vi "CreateARtoolkitHeader.vi"(8 "error in (no error)":errorcluster) -> (0 "error out":errorcluster, 1 "Starting Column of Each Variable":i32[](array[numeric]), 2 "Number of Columns":i32, 3 "header":string)   [LabVIEW 2016]
uses:
  <vilib>/GoldZinc Software/auzn custom VIs/CustomVI.lvlib
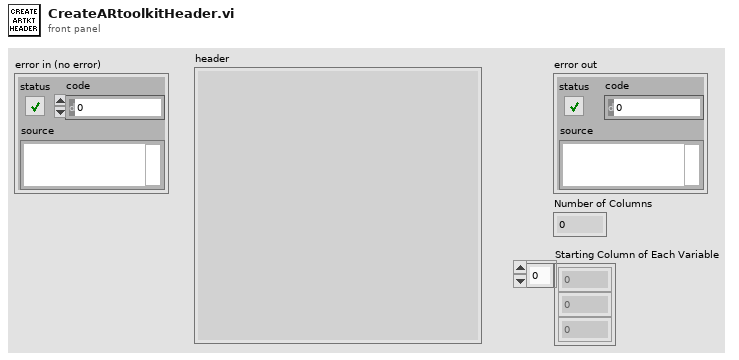
[diagram p1: front panel]
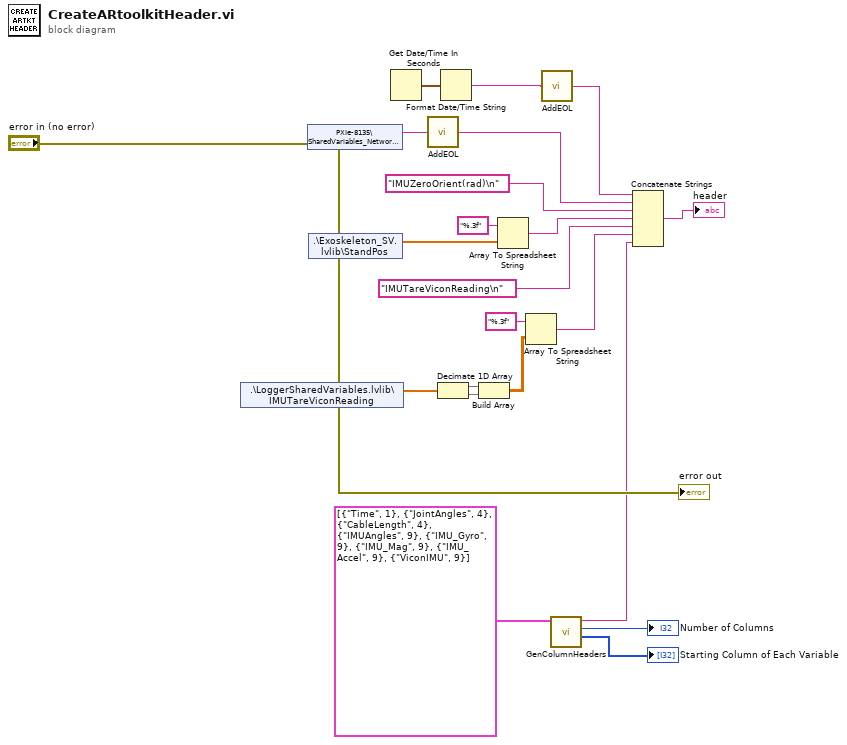
[diagram p0: block diagram]
diagram:
  n1 = shared-variable "PXIe-8135\\SharedVariables_Network.lvlib\\FileName"(error in="error in (no error)") -> (w21:string, error out=w13:errorcluster)
  n2 = shared-variable ".\\Exoskeleton_SV.lvlib\\StandPos"(error in=w13) -> (w16:dbl[], error out=w10:errorcluster)
  n3 = shared-variable ".\\LoggerSharedVariables.lvlib\\IMUTareViconReading"(error in=w10) -> (w4:dbl[], error out=→"error out":errorcluster)
  n4 = Get Date/Time In Seconds() -> (seconds since 1Jan1904=w24:timestamp)
  n5 = call <vilib>:"AddEOL.vi"("String in"=w21) -> ("String+\\n"=w12:string)
  n6 = Decimate 1D Array(w4) -> (w2:dbl[], w3:dbl[])
  n7 = Format Date/Time String(seconds (now)=w24) -> (date/time string=w20:string)  [unwired: 2 in]
  n8 = Build Array(w2, w3) -> (w1:dbl[][])
  n9 = Array To Spreadsheet String(array=w16, 3:"%.3f" ("format string")) -> (spreadsheet string=w15:string)  [unwired: 1 in]
  n10 = Array To Spreadsheet String(array=w1, 3:"%.3f" ("format string")) -> (spreadsheet string=w5:string)  [unwired: 1 in]
  n11 = call <vilib>:"AddEOL.vi"("String in"=w20) -> ("String+\\n"=w11:string)
  n12 = call "GenColumnHeaders.vi"("Array in"=cluster{string, i32}[] [{"Time", 1}, {"JointAngles", 4}, {"CableLength", 4}, {"IMUAngles", 9}, {"IMU_Gyro", 9}, {"IMU_Mag", 9}, {"IMU_Accel", 9}, {"ViconIMU", 9}] ("Array")) -> ("Starting Column of Each Variable"=→"Starting Column of Each Variable":i32[], "Total Number of Columns"=→"Number of Columns":i32, "String+\\n"=w7:string)  [unwired: 8 in]
  n13 = Concatenate Strings(w11, w12, "IMUZeroOrient(rad)\n" ("string"), w15, "IMUTareViconReading\n" ("string"), w5, w7) -> (→"header":string)
